vi "MM_RemoveControls.vi"(8 "error in (no error)":errorcluster, 11 "vi ref in":refnum<vi>) -> (0 "error out":errorcluster, 3 "vi ref out":refnum<vi>)   [LabVIEW 2012]
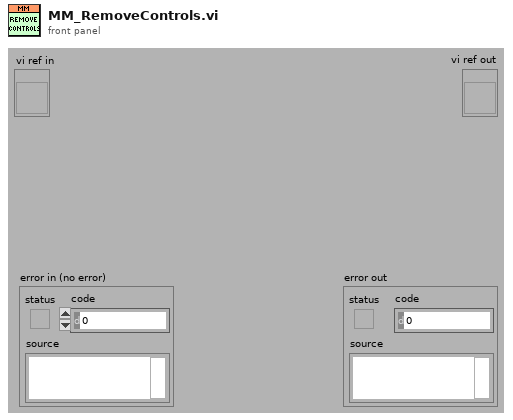
[diagram p1: front panel]
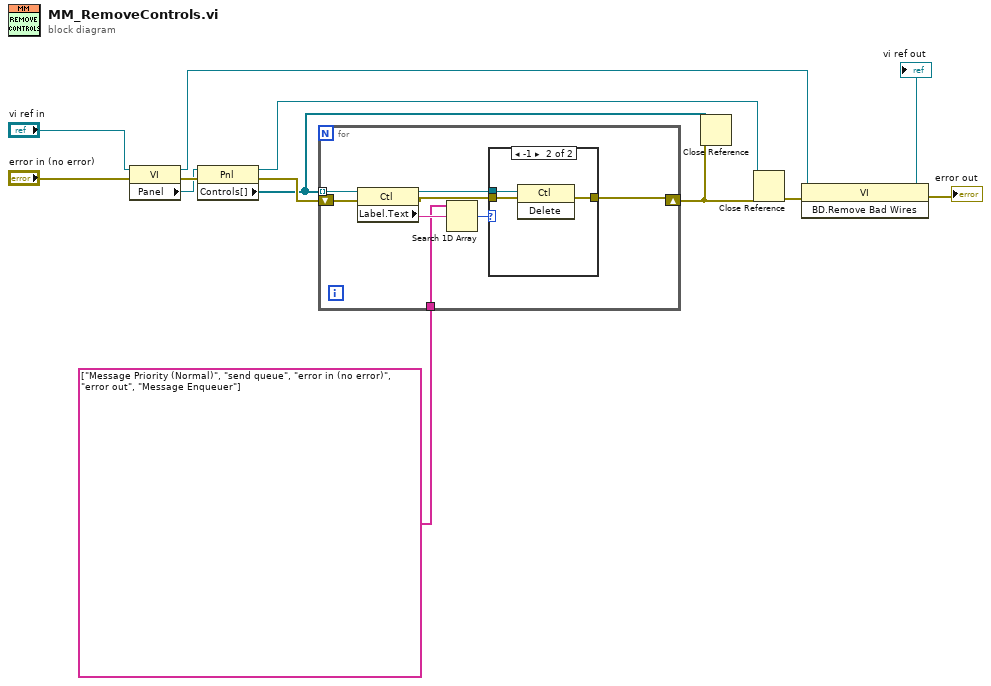
[diagram p0: block diagram]
diagram:
  n1 = property class="VI"(reference="vi ref in", error in="error in (no error)") -> (reference out=w7:refnum<vi>, error out=w11:errorcluster, "Panel"=w6:refnum<vi>)
  n2 = property class="Pnl"(reference=w6, error in=w11) -> (reference out=w2:refnum<vi>, error out=w9:errorcluster, "Controls[]"=w8:refnum<vi>[])
  n3 = for {
    tunnel: w8 -> [w21] mode=indexing
    tunnel: string[] ["Message Priority (Normal)", "send queue", "error in (no error)", "error out", "Message Enqueuer"] -> [w19]
    shift-right: [w14] -> w1
    shift-left: w9 -> [w15]
    n4 = property class="Ctl"(reference=w21, error in=w15) -> (reference out=w17:refnum<vi>, error out=w16:errorcluster, "Label.Text"=w20:string)
    n5 = Search 1D Array(1D array=w19, element=w20) -> (index of element=w18:i32)  [unwired: 1 in]
    n6 = case shown="-1" w18 {
      tunnel: w17 -> [_ w25]
      tunnel: w16 -> [w22 w24]
      tunnel: [w22 w23] -> w14
      frame 0, Default {
      }
      frame -1 {
        n7 = invoke class="Ctl" method="Delete"(reference=w25, error in=w24) -> (error out=w23:errorcluster)  [unwired: 1 in, 2 out]
      }
    }
  }
  n8 = Close Reference(reference=w8, error in (no error)=w1) -> ()  [unwired: 1 out]
  n9 = Close Reference(reference=w2, error in (no error)=w1) -> (error out=w3:errorcluster)
  n10 = invoke class="VI" method="BD.Remove Bad Wires"(reference=w7, error in=w3) -> (reference out=→"vi ref out":refnum<vi>, error out=→"error out":errorcluster)  [unwired: 1 in, 1 out]
